vi "Rapid Read_LeCroy_Done.vi"(0 "Digitizer ID Cluster.LeCroy VISA":refnum<visa-resource-name>, 1 "Motion Settings In":T1={"No Motion?"=FALSE, "Motion System"=enum."NI 735x", "Motion Bd ID"=1, "Motion Profile"="SMAC1", "# Axis"=1, "Reverse Z axis?"=TRUE, "SMAC Axis"=0, "scan pair"=enum."y-(x) scan", "RT fps"=6.0, "Steps per mm"=[1000, 1000, 1000, 1000], "Motor Parameters"={"velocity ct/s"=[10000.0, 10000.0, 10000.0, 50000.0], "accel ct/s^2"=[50000.0, 50000.0, 50000.0, 200000.0]}, "One Way Scan"=FALSE, "Reverse One Way Scan"=FALSE, "Global Position (mm)"=[], "Plane"=0, "Distance between\nscan lines (um)"=0.0, "Distance between\nscan planes (um)"=0.0, "number of scan planes"=1, "Total steps in line"=0, "Xtra plane\ndistance  (um)"=100, "Xtra planes "=1, "Add Axis"=FALSE, "overshoot cts"=200, "BKPT Shift"=0, "Scan Start Time (ms)"=0, "ESP VISA"="GPIB::1::INSTR", "3rd Axis"=1, "GL Ref Out"=refnum, "Galil Address"=""} {"3rd Axis" items=["x", "y", "z", "w"]; "Xtra planes" min=1; "Xtra plane\ndistance  (um)" min=0; "Distance between\nscan planes (um)" format="%.2f"; "Distance between\nscan lines (um)" format="%.2f"; "SMAC Axis" items=["None"=0, "Axis 1"=1, "Axis 2"=2, "Axis 3"=3, "Axis 4"=4, "Axis 5"=5, "Axis 6"=6, "Axis 7"=7, "Axis 8"=8, "Vector Space 1"=17, "Vector Space 2"=18, "Vector Space 3"=19, "Vector Space 4"=20]; "Motion Bd ID" min=1 max=32 step=1}, 9 "records":i32, 11 "error in":errorcluster, 14 "Pause?":bool) -> (6 "Reverse?":bool, 15 "error out":errorcluster)   [LabVIEW 2022 SP3]
uses:
  Motion Controllers/NI_controller/-NI_MotionRoutines/MotionParameters.ctl
  Motion Controllers/NI_controller/-NI_MotionRoutines/MotionSys.ctl
  Motion Controllers/-MotionRoutines/ScanAxis.ctl
  Motion Controllers/-MotionRoutines/3rdAxis.ctl
  Motion Controllers/Galil/Command Menu.ctl
  <vilib>/DAQmx/write.llb/DAQmx Write (Digital Bool 1Line 1Point).vi
  Motion Controllers/-MotionRoutines/MotionGlobals.vi
  <vilib>/DAQmx/miscellaneous.llb/DAQmx Fill In Error Info.vi
  <instrlib>/LeCroy Wave Series/LeCroy Wave Series.lvlib
panel:
  # "1-D and 2-D B scan settings"
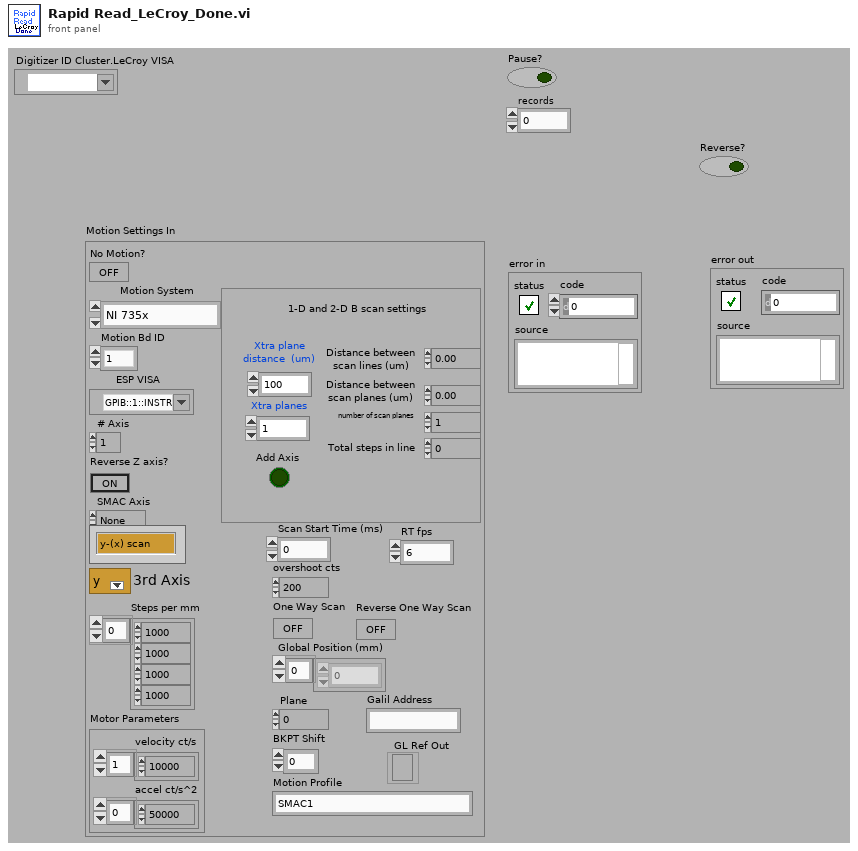
[diagram p1: front panel]
types:
  T1 = typedef "MotionParameters.ctl" = cluster{"No Motion?":bool, "Motion System":T2, "Motion Bd ID":u8, "Motion Profile":string, "# Axis":i8, "Reverse Z axis?":bool, "SMAC Axis":u16, "scan pair":T3, "RT fps":sgl, "Steps per mm":i32[], "Motor Parameters":cluster{"velocity ct/s":dbl[], "accel ct/s^2":dbl[]}, "One Way Scan":bool, "Reverse One Way Scan":bool, "Global Position (mm)":dbl[], "Plane":i32, "Distance between\nscan lines (um)":sgl, "Distance between\nscan planes (um)":sgl, "number of scan planes":i32, "Total steps in line":i32, "Xtra plane\ndistance  (um)":i32, "Xtra planes ":i32, "Add Axis":bool, "overshoot cts":i32, "BKPT Shift":i32, "Scan Start Time (ms)":u32, "ESP VISA":refnum<visa-resource-name>, "3rd Axis":T4, "GL Ref Out":refnum<k7>, "Galil Address":string}
  T2 = typedef "MotionSys.ctl" = enum16{"MM3000", "NI 735x", "Newport ESP", "No Motion Card", "Galil"}
  T3 = typedef "ScanAxis.ctl" = enum16{"y-(x) scan", "x-(y) scan", "z-(x) scan", "z-(y) scan", "y-(z) scan", "x-(z) scan", "w-(x) scan", "w-(y) scan", "w-(z) scan", "x-(w) scan", "y-(w) scan", "z-(w) scan"}
  T4 = typedef "3rdAxis.ctl" = u16
  T5 = typedef "Command Menu.ctl" = enum16{"CommandPassThrough", "Abort Motion", "Define Pos", "Velocity", "Acceleration", "Deceleration", "Position Rel", "Postion Abs", "Begin Move", "After Move", "Home", "KI", "KD", "KP", "IL", "Config I/O", "Set Bit", "Clear Bit", "Motor Off", "Moto On", "Status", "Execute", "Halt Execute", "HX Status", "Tell Velocity", "Check Motion", "BreakPoint", "Tell Position", "Current Code Line", "Tell Switches", "OC Force On", "OC Off", "Pos Soft Limit", "Rev Soft Limit"}
  T6 = typedef "Var" = u8
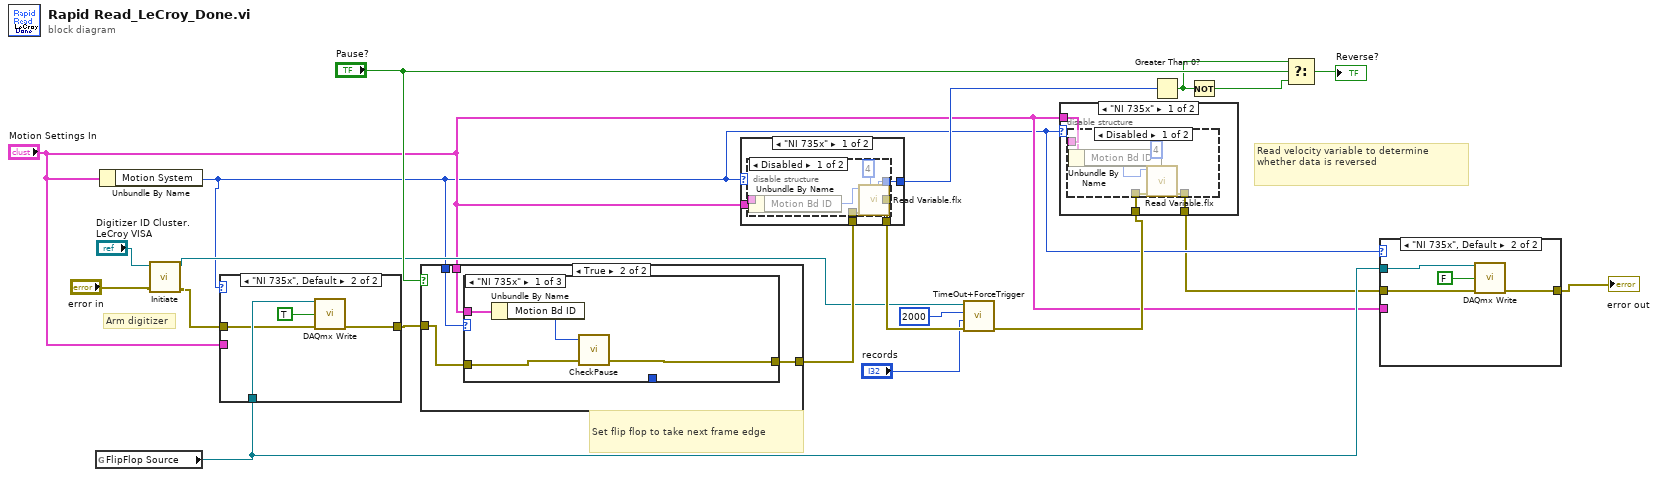
[diagram p0: block diagram]
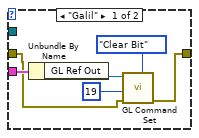
[diagram p2: hidden frame]
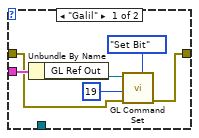
[diagram p3: hidden frame]
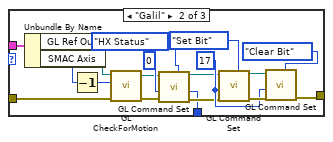
[diagram p9: hidden frame]
diagram:
  # "Arm digitizer"
  # "Set flip flop to take next frame edge"
  # "Read velocity variable to determine whether data is reversed"
  n1 = global read "MotionGlobals.vi" "FlipFlop Source"() -> (w5:refnum<k21>)
  n2 = Unbundle By Name("Motion Settings In") -> ("Motion System"=w3:T2)
  n3 = call <instrlib>:"Initiate.vi"("error in (no error)"="error in", "VISA resource name"="Digitizer ID Cluster.LeCroy VISA") -> ("error out"=w13:errorcluster, "VISA resource name out"=w7:refnum<visa-resource-name>)  [unwired: 8 in]
  n4 = case shown="\"NI 735x\", Default" w3 {
    tunnel: [w22 w29] -> w19
    tunnel: w5 -> [_ w28]
    tunnel: w13 -> [w21 w27]
    tunnel: "Motion Settings In" -> [w23 _]
    frame "Galil" {
      n5 = Unbundle By Name(w23) -> ("GL Ref Out"=w26:refnum<k7>)
      n6 = call "GL Command Set.vi"("Command"=Command_Menu."Set Bit", "error in (no error)"=w21, "Value"=19, "Galil.IGalil"=w26) -> ("error out"=w22:errorcluster)  [unwired: 3 in, 4 out]
    }
    frame "NI 735x", Default {
      n7 = call-poly <vilib>:"DAQmx Write.vi"("task/channels in"=w28, "data"=TRUE ("stop (T)"), "error in"=w27) -> ("error out"=w29:errorcluster)  [unwired: 10 in, 2 out]
    }
  }
  n8 = case shown="True" "Pause?" {
    tunnel: w19 -> [w31 w35]
    tunnel: [w31 w32] -> w11
    tunnel: w3 -> [_ w34]
    tunnel: "Motion Settings In" -> [_ w33]
    frame False {
    }
    frame True {
      n9 = case shown="\"NI 735x\"" w34 {
        tunnel: [w39 w53 w58] -> w32
        tunnel: w35 -> [w38 w56 w58]
        tunnel: w33 -> [w37 w49 _]
        tunnel: [_ w40 _] -> _
        frame "NI 735x" {
          n10 = Unbundle By Name(w37) -> ("Motion Bd ID"=w36:u8)
          n11 = call "CheckPause.vi"("error in"=w38, "Motion Board ID"=w36) -> ("error out"=w39:errorcluster)  [unwired: 3 in]
        }
        frame "Galil" {
          w50 = 17 ("Value")
          n12 = Unbundle By Name(w49) -> ("GL Ref Out"=w48:refnum<k7>, "SMAC Axis"=w47:u16)
          n13 = Decrement(x=w47) -> (x-1=w57:u16)
          n14 = call "GL CheckForMotion.vi"("error in"=w56, "Axis"=w57, "Refnum in"=w48) -> ("error out"=w44:errorcluster, "Refnum out"=w41:refnum<k7>)  [unwired: 6 in, 1 out]
          n15 = call "GL Command Set.vi"("Command"=Command_Menu."HX Status", "error in (no error)"=w44, "Value"=0, "Galil.IGalil"=w41) -> ("error out"=w43:errorcluster, "Response#"=w40:i32, "ref out"=w42:refnum<k7>)  [unwired: 3 in, 2 out]
          n16 = call "GL Command Set.vi"("Command"=Command_Menu."Set Bit", "error in (no error)"=w43, "Value"=w50, "Galil.IGalil"=w42) -> ("error out"=w54:errorcluster, "ref out"=w51:refnum<k7>)  [unwired: 3 in, 3 out]
          n17 = call "GL Command Set.vi"("Command"=Command_Menu."Clear Bit", "error in (no error)"=w54, "Value"=w50, "Galil.IGalil"=w51) -> ("error out"=w53:errorcluster)  [unwired: 3 in, 4 out]
        }
        frame "No Motion Card", Default {
        }
      }
    }
  }
  n18 = case shown="\"NI 735x\"" w3 {
    tunnel: [w62 w69] -> w10
    tunnel: [w61 _] -> w20
    tunnel: w11 -> [w60 w69]
    tunnel: "Motion Settings In" -> [w59 _]
    frame "NI 735x" {
      n19 = disable-structure shown="Disabled" {
        disable-tunnel: [w67 _] -> w62
        disable-tunnel: [w66 _] -> w61
        disable-tunnel: w60 -> [w65 _]
        disable-tunnel: w59 -> [w64 _]
        frame Disabled {
          n20 = Unbundle By Name(w64) -> ("Motion Bd ID"=w63:u8)
          n21 = call <vilib>:"Read Variable.flx"("Var"=T6 4, "error in (no error)"=w65, "Board ID"=w63) -> ("error out"=w67:errorcluster, "Output"=w66:i32)  [unwired: 1 in, 4 out]
        }
        frame Enabled {
        }
      }
    }
    frame "No Motion Card", Default {
    }
  }
  n22 = call "TimeOut+ForceTrigger.vi"("error in (no error)"=w10, "lines per plane mod"="records", "Timeout (10000 ms)"=u32 2000, "VISA resource name"=w7) -> ("error out"=w8:errorcluster)  [unwired: 4 in, 3 out]
  n23 = case shown="\"NI 735x\"" w3 {
    tunnel: w8 -> [w72 w78]
    tunnel: [w71 w78] -> w2
    tunnel: "Motion Settings In" -> [w70 _]
    frame "NI 735x" {
      n24 = disable-structure shown="Disabled" {
        disable-tunnel: w72 -> [w76 _]
        disable-tunnel: [w75 _] -> w71
        disable-tunnel: w70 -> [w74 _]
        frame Disabled {
          n25 = Unbundle By Name(w74) -> ("Motion Bd ID"=w73:u8)
          n26 = call <vilib>:"Read Variable.flx"("Var"=T6 4, "error in (no error)"=w76, "Board ID"=w73) -> ("error out"=w75:errorcluster)  [unwired: 1 in, 5 out]
        }
        frame Enabled {
        }
      }
    }
    frame "No Motion Card", Default {
    }
  }
  n27 = Greater Than 0?(x=w20) -> (x > 0?=w17:bool)
  n28 = Not(x=w17) -> (.not. x?=w16:bool)
  n29 = Select(t=w17, s="Pause?", f=w16) -> (s? t:f=→"Reverse?":bool)
  n30 = case shown="\"NI 735x\", Default" w3 {
    tunnel: [w80 w87] -> w1
    tunnel: w2 -> [w79 w86]
    tunnel: "Motion Settings In" -> [w81 _]
    tunnel: w5 -> [_ w85]
    frame "Galil" {
      n31 = Unbundle By Name(w81) -> ("GL Ref Out"=w84:refnum<k7>)
      n32 = call "GL Command Set.vi"("Command"=Command_Menu."Clear Bit", "error in (no error)"=w79, "Value"=19, "Galil.IGalil"=w84) -> ("error out"=w80:errorcluster)  [unwired: 3 in, 4 out]
    }
    frame "NI 735x", Default {
      n33 = call-poly <vilib>:"DAQmx Write.vi"("task/channels in"=w85, "data"=FALSE ("stop (T)"), "error in"=w86) -> ("error out"=w87:errorcluster)  [unwired: 10 in, 2 out]
    }
  }
  "error out" <- w1
